vi "Get Value of LabVIEW Array.vi"(1 "LabVIEW Array":refnum<vi>, 3 "error in (no error)":errorcluster) -> (7 "JSON Tree Array":variant, 10 "error out":errorcluster)   [LabVIEW 2013, in "i3-json.lvlib"]
doc: "This VI takes a JSON Node (all types besides JSON Object) and assigns the value to the LabVIEW Base Type of compatible reference.\n\nIf the LabVIEW base type is an array of boolean, numeric, or string this function will attempt to check if a JSON Array type will map"
uses:
  i3-json.lvlib
  JSON Types/JSON Type.ctl
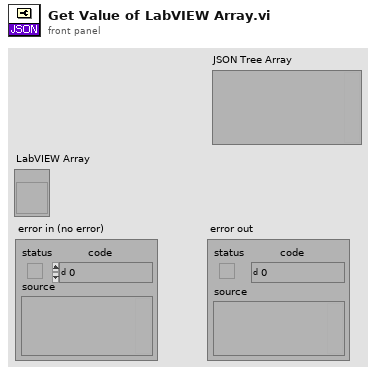
[diagram p1: front panel]
types:
  T1 = typedef "i3-json.lvlib/JSON Type.ctl" = enum8{"JSON Compatible", "JSON Array", "JSON Object", "JSON Null", "Double", "String", "Boolean", "Unknown", "Data JSON string"}
  T2 = enum8{"Enabled", "Disabled", "Disabled and Grayed Out"}
  T3 = typedef "Type Enum.ctl" = enum8{"Void", "I8", "I16", "I32", "I64", "U8", "U16", "U32", "U64", "Single Float", "Double Float", "Extended Float", "Single Complex", "Double Complex", "Extended Complex", "Enum I8 NEVER", "Enum I16 NEVER", "Enum I32 NEVER", "Enum I64 NEVER", "Enum U8", "Enum U16", "Enum U32", "Enum U64", "Single Float With Unit", "Double Float With Unit", "Extended Float With Unit", "Single Complex With Unit", "Double Complex With Unit", "Extended Complex With Unit", "boolU16", "Boolean", "String", "Handle", "Path", "Picture", "C String", "Pascal String", "Tag", "SubString", "Array", "SubArray", "Cluster", "Numeric Cluster", "Variant", "LV Variant", "Measure Data (waveform)", "Refnum", "ExtData", "function", "Typedef", "Poly VI", "bad wire", "LabVIEW Class Instance"}
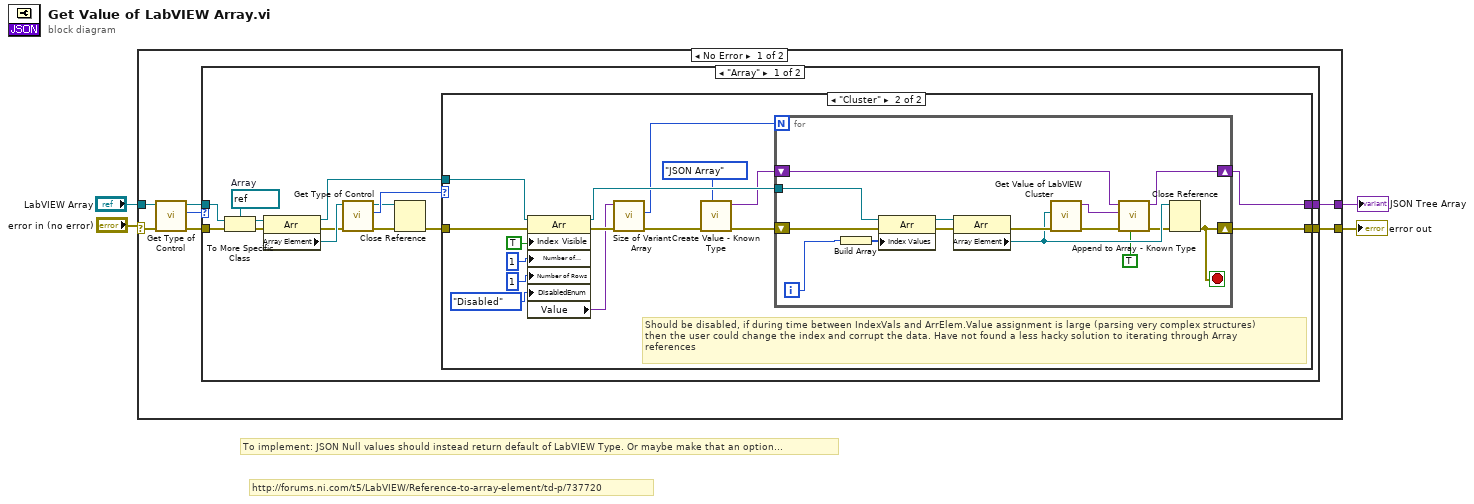
[diagram p0: block diagram]
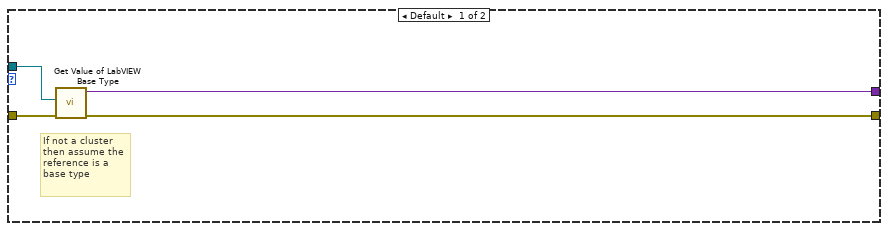
[diagram p2: hidden frame]
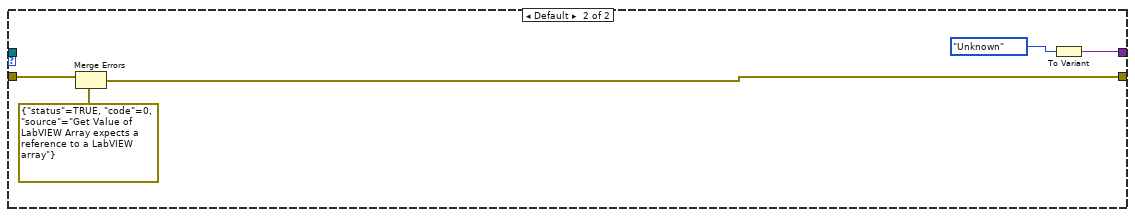
[diagram p3: hidden frame]
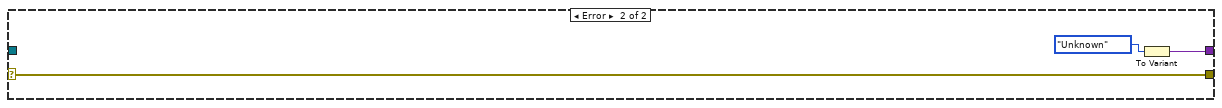
[diagram p4: hidden frame]
diagram:
  # "http://forums.ni.com/t5/LabVIEW/Reference-to-array-element/td-p/737720"
  # "To implement: JSON Null values should instead return default of LabVIEW Type. Or maybe make that an option..."
  n1 = case shown="No Error" "error in (no error)" {
    selector: "error in (no error)" -> [w11 w68]
    tunnel: "LabVIEW Array" -> [w10 _]
    tunnel: [w6 w68] -> w2
    tunnel: [w5 w67] -> w1
    frame No Error {
      n2 = call <vilib>:"Get Type of Control.vi"("error in (no error)"=w11, "Control Ref In"=w10) -> ("error out"=w7:errorcluster, "Type Enum"=w9:T3, "Control Ref Out"=w8:refnum<vi>)  [unwired: 7 in]
      n3 = case shown="\"Array\"" w9 {
        tunnel: w8 -> [w24 _]
        tunnel: w7 -> [w25 w65]
        tunnel: [w18 w64] -> w6
        tunnel: [w12 w62] -> w5
        frame "Array" {
          w19 = refnum<vi> refnum  # Array
          n4 = To More Specific Class(target class=w19, reference=w24, error in=w25) -> (specific class reference=w17:refnum<vi>, error out=w23:errorcluster)
          n5 = property class="Arr"(reference=w17, error in=w23) -> (reference out=w13:refnum<vi>, error out=w21:errorcluster, "Array Element"=w22:refnum<vi>)
          n6 = call <vilib>:"Get Type of Control.vi"("error in (no error)"=w21, "Control Ref In"=w22) -> ("error out"=w16:errorcluster, "Type Enum"=w20:T3, "Control Ref Out"=w14:refnum<vi>)  [unwired: 7 in]
          n7 = Close Reference(reference=w14, error in (no error)=w16) -> (error out=w15:errorcluster)
          n8 = case shown="\"Cluster\"" w20 {
            tunnel: w15 -> [w29 w38]
            tunnel: w13 -> [w28 w41]
            tunnel: [w27 w39] -> w18
            tunnel: [w26 w30] -> w12
            frame Default {
              # "If not a cluster then assume the reference is a base type"
              n9 = call "Get Value of LabVIEW Base Type.vi"("LabVIEW Base Type"=w28, "error in (no error)"=w29) -> ("JSON Tree Out"=w26:variant, "error out"=w27:errorcluster)  [unwired: 7 in]
            }
            frame "Cluster" {
              # "Should be disabled, if during time between IndexVals and ArrElem.Value assignment is large (parsing very complex structures)\nthen the user could change the index and corrupt the data. Have not found a less hacky solution to iterating through Array\nreferences"
              n10 = property class="Arr"(reference=w41, error in=w38, "Index Visible"=TRUE, "Number of Columns"=u32 1, "Number of Rows"=u32 1, "DisabledEnum"=T2."Disabled" ("Disabled")) -> (reference out=w40:refnum<vi>, error out=w37:errorcluster, "Value"=w36:variant)
              n11 = call "Size of Variant Array.vi"("error in (no error)"=w37, "LabVIEW Array In"=w36) -> ("error out"=w33:errorcluster, "Size of Array"=w35:u32)  [unwired: 8 in]
              n12 = call "Create Value - Known Type.vi"("JSON Type"=JSON_Type."JSON Array", "error in (no error)"=w33) -> ("error out"=w34:errorcluster, "JSON Tree"=w31:variant)  [unwired: 8 in]
              n13 = for {
                N: w35 -> [_]
                tunnel: w40 -> [w60]
                shift-right: [w57] -> w30
                shift-left: w31 -> [w56]
                shift-right: [w46] -> w39
                shift-left: w34 -> [w58]
                i -> [w59]
                stop <- w46 stop-if-true
                n14 = Build Array(w59) -> (w55:i32[])
                n15 = property class="Arr"(reference=w60, error in=w58, "Index Values"=w55) -> (reference out=w54:refnum<vi>, error out=w53:errorcluster)
                n16 = property class="Arr"(reference=w54, error in=w53) -> (error out=w52:errorcluster, "Array Element"=w51:refnum<vi>)  [unwired: 1 out]
                n17 = call "Get Value of LabVIEW Cluster.vi"("error in (no error)"=w52, "LabVIEW Cluster"=w51) -> ("error out"=w49:errorcluster, "JSON Tree Object Out"=w48:variant)  [unwired: 8 in]
                n18 = call "Append to Array - Known Type.vi"("Add Parameter as JSON Tree?"=TRUE, "error in (no error)"=w49, "Value"=w48, "JSON Tree in (JSON Array)"=w56) -> ("error out"=w50:errorcluster, "JSON Tree out (JSON Array)"=w57:variant)  [unwired: 6 in]
                n19 = Close Reference(reference=w51, error in (no error)=w50) -> (error out=w46:errorcluster)
              }
            }
          }
        }
        frame Default {
          n20 = Merge Errors(w65, errorcluster {"status"=TRUE, "code"=0, "source"="Get Value of LabVIEW Array expects a reference to a LabVIEW array"} ("error in")) -> (w64:errorcluster)
          n21 = To Variant(anything=JSON_Type."Unknown" ("JSON Type")) -> (Variant=w62:variant)
        }
      }
    }
    frame Error {
      n22 = To Variant(anything=JSON_Type."Unknown" ("JSON Type")) -> (Variant=w67:variant)
    }
  }
  "JSON Tree Array" <- w1
  "error out" <- w2
